vi "subGenerateIncrementBuildFileName.vi"(11 "Path in":path) -> (3 "Path out":path)   [LabVIEW 2019, in "SolutionBuilder.lvlib" / "SolutionBuilder.lvclass"]
uses:
  SolutionBuilder.lvclass
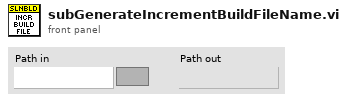
[diagram p1: front panel]
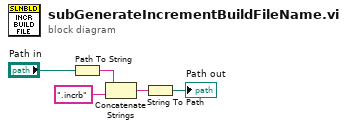
[diagram p0: block diagram]
diagram:
  n1 = Path To String(path="Path in") -> (string=w2:string)
  n2 = Concatenate Strings(w2, ".incrb" ("string")) -> (w4:string)
  n3 = String To Path(string=w4) -> (path=→"Path out":path)
